vi "DriveStraight.vi"(4 "EncData":T1, 6 "FirstTime?":bool, 7 "GyroData":T2, 8 "Decel?":bool, 9 "Accel?":bool, 10 "MinPwr":dbl, 11 "MaxPwr":dbl) -> (0 "RightOut":dbl, 3 "LeftOut":dbl)   [LabVIEW 2017]
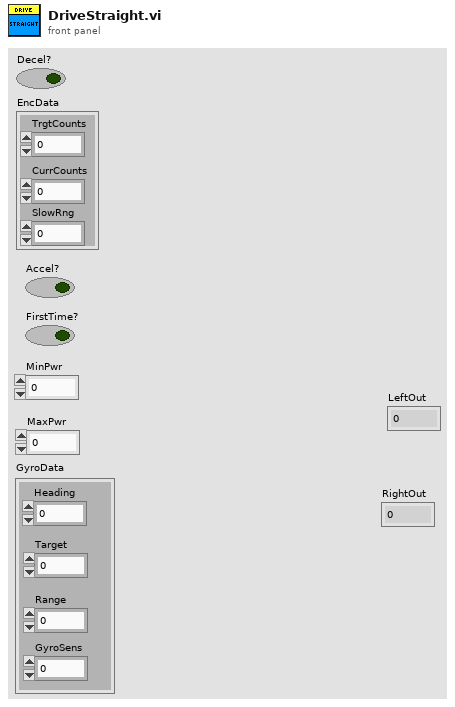
[diagram p1: front panel]
types:
  T1 = cluster{"TrgtCounts":i32, "CurrCounts":dbl, "SlowRng":dbl}
  T2 = cluster{"Heading":dbl, "Target":dbl, "Range":dbl, "GyroSens":dbl}
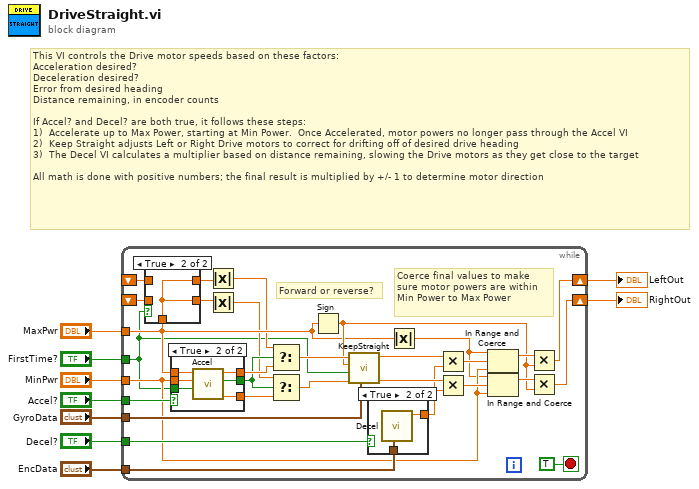
[diagram p0: block diagram]
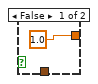
[diagram p3: hidden frame]
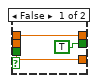
[diagram p4: hidden frame]
diagram:
  # "This VI controls the Drive motor speeds based on these factors:\nAcceleration desired?\nDeceleration desired?\nError from desired heading\nDistance remaining, in encoder counts\n\nIf Accel? and Decel? are both true, it follows these steps:\n1)  Accelerate up to Max Power, starting at Min Power.  Once Accelerated, motor powers no longer pass through the Accel VI\n2)  Keep Straight adjusts Left or Right Drive motors to correct for drifting off of desired drive heading\n3)  The Decel VI calculates a multiplier based on distance remaining, slowing the Drive motors as they get close to the target\n\nAll math is done with positive numbers; the final result is multiplied by +/- 1 to determine motor direction"
  n1 = while {
    tunnel: "MaxPwr" -> [w16]
    tunnel: "FirstTime?" -> [w10]
    shift-right: [w18] -> w8
    shift-left: _ -> [w30]
    shift-right: [w19] -> w7
    shift-left: _ -> [w31]
    tunnel: "MinPwr" -> [w17]
    tunnel: "Accel?" -> [w38]
    tunnel: "GyroData" -> [w29]
    tunnel: "Decel?" -> [w33]
    tunnel: "EncData" -> [w32]
    stop <- TRUE stop-if-true
    # "Coerce final values to make sure motor powers are within Min Power to Max Power"
    # "Forward or reverse?"
    n2 = case shown="True" w10 {
      tunnel: w31 -> [w41 _]
      tunnel: [w41 w42] -> w12
      tunnel: [w40 w42] -> w14
      tunnel: w30 -> [w40 _]
      tunnel: w16 -> [_ w42]
      frame False {
      }
      frame True {
      }
    }
    n3 = case shown="True" w38 {
      tunnel: [w46 w53] -> w37
      tunnel: [w46 w52] -> w36
      tunnel: [TRUE ("Acceled?") w51] -> w28
      tunnel: w10 -> [_ w50]
      tunnel: w16 -> [w46 w49]
      tunnel: w17 -> [_ w48]
      frame False {
      }
      frame True {
        n4 = call "Accel.vi"("FirstTime?"=w50, "MinPwr"=w48, "MaxPwr"=w49) -> ("RightSpdOut"=w52:dbl, "Acceled?"=w51:bool, "LeftSpdOut"=w53:dbl)  [unwired: 6 in]
      }
    }
    n5 = Absolute Value(x=w12) -> (abs(x)=w11:dbl)
    n6 = Absolute Value(x=w14) -> (abs(x)=w13:dbl)
    n7 = Select(t=w11, s=w28, f=w37) -> (s? t:f=w35:dbl)
    n8 = Select(t=w13, s=w28, f=w36) -> (s? t:f=w34:dbl)
    n9 = Sign(1:w16) -> (0:w20:dbl)
    n10 = call "KeepStraight.vi"("GyroData"=w29, "RightSpdIn"=w34, "FirstTime?"=w10, "MtrDir"=w20, "LeftSpdIn"=w35) -> ("RightSpdOut"=w26:dbl, "LeftSpdOut"=w27:dbl)  [unwired: 5 in]
    n11 = case shown="True" w33 {
      tunnel: [1.0 ("SpdMult") w45] -> w25
      tunnel: w32 -> [_ w44]
      frame False {
      }
      frame True {
        n12 = call "Decel.vi"("EncData"=w44) -> ("SpdMult"=w45:dbl)  [unwired: 10 in]
      }
    }
    n13 = Absolute Value(x=w16) -> (abs(x)=w15:dbl)
    n14 = Multiply(x=w27, y=w25) -> (x*y=w24:dbl)
    n15 = Multiply(x=w26, y=w25) -> (x*y=w23:dbl)
    n16 = In Range and Coerce(upper limit=w15, x=w24, lower limit=w17) -> (coerced(x)=w22:dbl)  [unwired: 1 out]
    n17 = In Range and Coerce(upper limit=w15, x=w23, lower limit=w17) -> (coerced(x)=w21:dbl)  [unwired: 1 out]
    n18 = Multiply(x=w22, y=w20) -> (x*y=w19:dbl)
    n19 = Multiply(x=w21, y=w20) -> (x*y=w18:dbl)
  }
  "LeftOut" <- w7
  "RightOut" <- w8
